vi "face getcolumn.vi"(7 "reverse? (F)":bool, 8 "error in (no error)":errorcluster, 9 "slice number":u8, 11 "face in":T2) -> (0 "error out":errorcluster, 3 "slice":T1)   [LabVIEW 2011]
uses:
  Typedef/face.ctl
  Typedef/slice.ctl
  Typedef/slice type.ctl
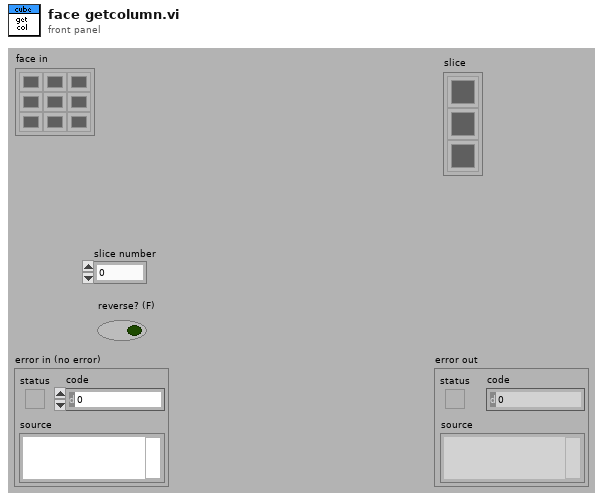
[diagram p1: front panel]
types:
  T1 = typedef "slice.ctl" = u32[]
  T2 = typedef "face.ctl" = u32[][]
  T3 = typedef "slice type.ctl" = enum16{"row", "col"}
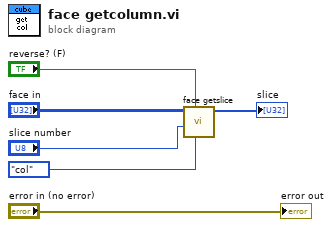
[diagram p0: block diagram]
diagram:
  n1 = call "face getslice.vi"("slice type"=slice_type."col", "reverse? (F)"="reverse? (F)", "slice number"="slice number", "face in"="face in") -> ("slice"=→"slice":T1)  [unwired: 6 in, 1 out]
  "error out" <- "error in (no error)"
